vi "get all tags in collection.vi"(8 "error in":errorcluster, 11 "tag collection in":refnum<class "data bus tag collection.lvclass">) -> (0 "error out":errorcluster, 2 "tags":refnum<class "data bus tag description.lvclass">[](array[class]), 3 "tag collection out":refnum<class "data bus tag collection.lvclass">)   [LabVIEW 2013, in "data bus tag collection.lvclass"]
uses:
  data bus tag collection.lvclass
  tag/data bus tag description.lvclass
  data bus tag collection.lvclass/data bus tag collection.ctl
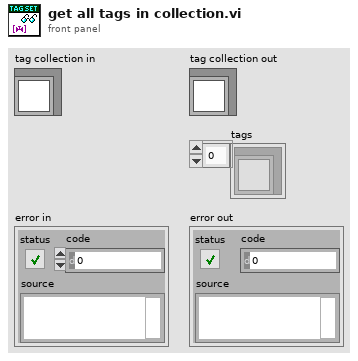
[diagram p1: front panel]
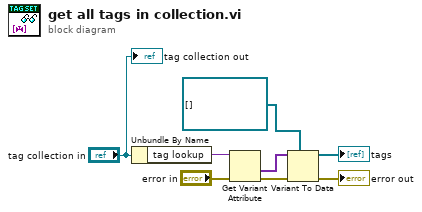
[diagram p0: block diagram]
diagram:
  n1 = Unbundle By Name("tag collection in") -> ("tag lookup"=w7:variant)
  n2 = Get Variant Attribute(Variant=w7, error in="error in") -> (values=w6:variant[], error out=w3:errorcluster)  [unwired: 2 in, 2 out]
  n3 = Variant To Data(error in=w3, type=refnum<class "data bus tag description.lvclass">[] [] ("tags"), Variant=w6) -> (data=→"tags":refnum<class "data bus tag description.lvclass">[], error out=→"error out":errorcluster)
  "tag collection out" <- "tag collection in"
